vi "SUB_SFCS_SendResult.vi"(1 "ErrorCode":string, 2 "PASS_Fail (1/0)":i8) -> (0 "Sent OK ?":bool)   [LabVIEW 2011]
uses:
  Instance           4 27Saved   SUB_SFCS_SendResult .vi
  Instance           7 27Saved   SUB_SFCS_SendResult .vi
  Instance           8 27Saved   SUB_SFCS_SendResult .vi
  Instance          10 27Saved   SUB_SFCS_SendResult .vi
  Instance          11 27Saved   SUB_SFCS_SendResult .vi
  Instance          14 27Saved   SUB_SFCS_SendResult .vi
  Instance          15 27Saved   SUB_SFCS_SendResult .vi
  data/MCSDLL.dll
panel:
  out "output param":string
  out "SFCS System Enable":string
  out "OperatorID":string
  out "Line":string
  out "SN":string
  out "Station":string
  out "STAGE":string
  out "SFCS_IP":string
  in  "URL":string
  # "Send Result SFCS_Complete"
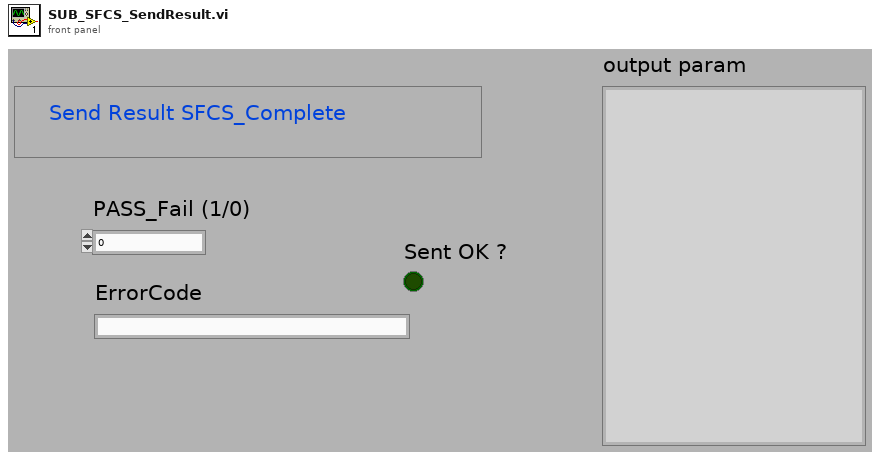
[diagram p1: front panel]
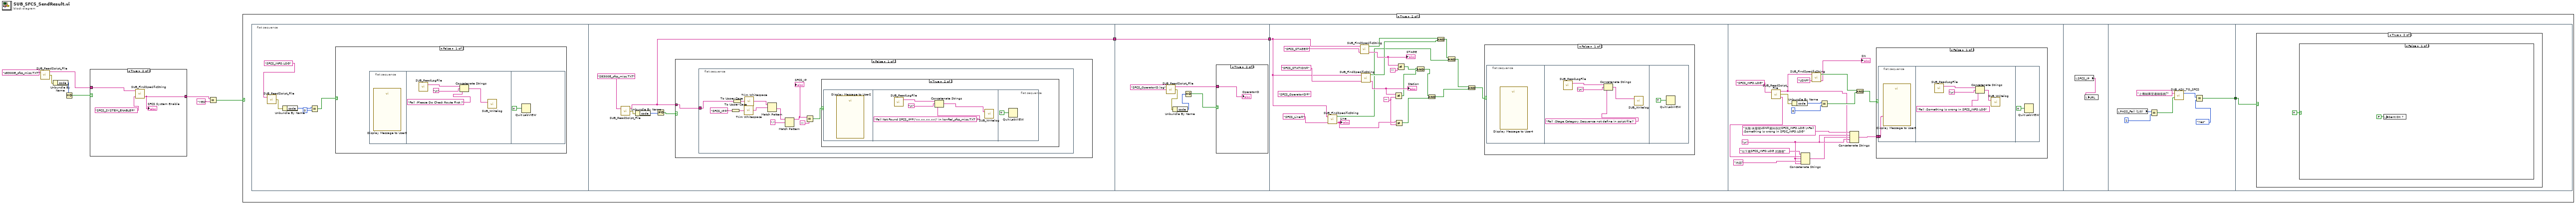
[diagram p0: block diagram]
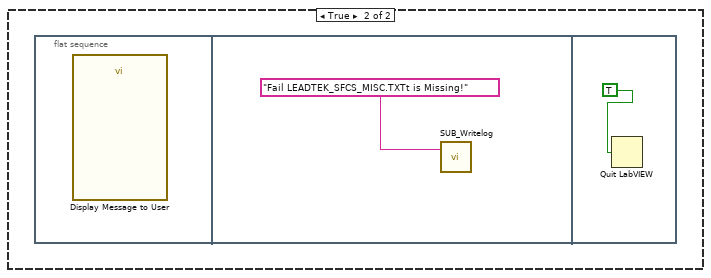
[diagram p5: hidden frame]
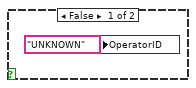
[diagram p6: hidden frame]
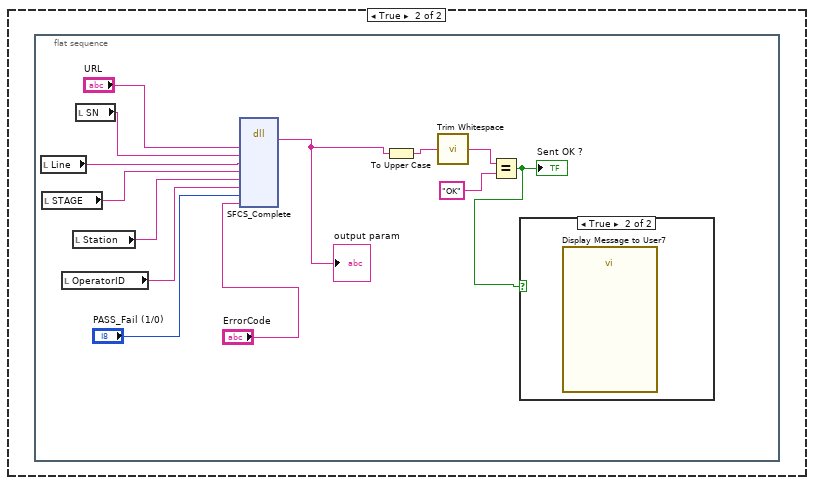
[diagram p10: hidden frame]
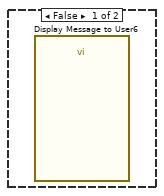
[diagram p11: hidden frame]
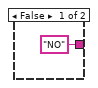
[diagram p12: hidden frame]
diagram:
  n1 = call "SUB_ReadScript_File.vi"("Script FileName"="s8300E_sfcs_misc.TXT") -> ("text"=w2:string, "error out"=w8:errorcluster)  [unwired: 1 in, 1 out]
  n2 = Unbundle By Name(w8) -> ("code"=w7:i32)
  n3 = Equal To 0?(x=w7) -> (x = 0?=w6:bool)
  n4 = case shown="True" w6 {
    tunnel: w2 -> [_ w12]
    tunnel: ["NO" ("before \"; \" string") w10] -> w4
    frame False {
    }
    frame True {
      n5 = call "SUB_FindSpecificString.vi"("Find this String"="SFCS_SYSTEM_ENABLE=", "String data"=w12) -> ("before \"; \" string"=w10:string)  [unwired: 2 in, 1 out]
      "SFCS System Enable" <- w10
    }
  }
  n6 = Equal?(x=w4, y="YES") -> (x = y?=w5:bool)
  n7 = case shown="True" w5 {
    frame False {
    }
    frame True {
      n8 = flat-sequence {
        tunnel: [w27] -> w14
        tunnel: w14 -> [w55]
        tunnel: [w55] -> w13
        tunnel: w13 -> [w73]
        tunnel: [w111] -> w15
        tunnel: w15 -> [w115]
        frame #0 {
          n9 = call "SUB_ReadScript_File.vi"("Script FileName"="SFCS_INFO.LOG" ("Search Filename in Folder")) -> ("error out"=w20:errorcluster)  [unwired: 1 in, 2 out]
          n10 = Unbundle By Name(w20) -> ("code"=w19:i32)
          n11 = Equal?(x=w19, y=0) -> (x = y?=w16:bool)
          n12 = case shown="False" w16 {
            frame False {
              n13 = flat-sequence {
                frame #0 {
                  n14 = call "Display Message to User3"() -> ()  [unwired: 10 in, 2 out]
                }
                frame #1 {
                  n15 = call "SUB_ReadLogFile.vi"() -> ("text"=w24:string)  [unwired: 2 in, 1 out]
                  n16 = Concatenate Strings(w24, "\n", "Fail :Please Do Check Route First !" ("Pass/Fail")) -> (w21:string)
                  n17 = call "SUB_Writelog.vi"("Pass/Fail"=w21) -> ()  [unwired: 2 in]
                }
                frame #2 {
                  n18 = Quit LabVIEW(quit? (T)=TRUE) -> ()
                }
              }
            }
            frame True {
            }
          }
        }
        frame #1 {
          n19 = call "SUB_ReadScript_File.vi"("Script FileName"="S8300E_sfcs_misc.TXT") -> ("text"=w27:string, "error out"=w30:errorcluster)  [unwired: 1 in, 1 out]
          n20 = Unbundle By Name(w30) -> ("code"=w29:i32)
          n21 = Not Equal To 0?(x=w29) -> (x != 0?=w28:bool)
          n22 = case shown="False" w28 {
            tunnel: w27 -> [w31 _]
            frame False {
              n23 = flat-sequence {
                tunnel: w31 -> [w37]
                frame #0 {
                  n24 = To Upper Case(1:"SFCS_IP=" ("string")) -> (0:w41:string)
                  n25 = To Upper Case(1:w37) -> (0:w42:string)
                  n26 = call <vilib>:"Trim Whitespace.vi"("string"=w41) -> ("trimmed string"=w39:string)  [unwired: 1 in]
                  n27 = call <vilib>:"Trim Whitespace.vi"("string"=w42) -> ("trimmed string"=w38:string)  [unwired: 1 in]
                  n28 = Match Pattern(string=w38, regular expression=w39) -> (after substring=w36:string)  [unwired: 1 in, 3 out]
                  n29 = Match Pattern(string=w36, regular expression=";") -> (before substring=w34:string)  [unwired: 1 in, 3 out]
                  "SFCS_IP" <- w34
                  n30 = Equal?(x=w34, y="") -> (x = y?=w32:bool)
                  n31 = case shown="True" w32 {
                    frame False {
                    }
                    frame True {
                      n32 = flat-sequence {
                        frame #0 {
                          n33 = call "Display Message to User2"() -> ()  [unwired: 10 in, 2 out]
                        }
                        frame #1 {
                          n34 = call "SUB_ReadLogFile.vi"() -> ("text"=w46:string)  [unwired: 2 in, 1 out]
                          n35 = Concatenate Strings(w46, "\n", "Fail Not Found SFCS_IP=\"xx.xx.xx.xx\" in konftel_sfcs_misc.TXT !" ("Pass/Fail")) -> (w43:string)
                          n36 = call "SUB_Writelog.vi"("Pass/Fail"=w43) -> ()  [unwired: 2 in]
                        }
                        frame #2 {
                          n37 = Quit LabVIEW(quit? (T)=TRUE) -> ()
                        }
                      }
                    }
                  }
                }
              }
            }
            frame True {
              n38 = flat-sequence {
                frame #0 {
                  n39 = call "Display Message to User"() -> ()  [unwired: 10 in, 2 out]
                }
                frame #1 {
                  n40 = call "SUB_Writelog.vi"("Pass/Fail"="Fail LEADTEK_SFCS_MISC.TXTt is Missing!") -> ()  [unwired: 2 in]
                }
                frame #2 {
                  n41 = Quit LabVIEW(quit? (T)=TRUE) -> ()
                }
              }
            }
          }
        }
        frame #2 {
          n42 = call "SUB_ReadScript_File.vi"("Script FileName"="SFCS_OperatorID.log" ("name or relative path")) -> ("text"=w50:string, "error out"=w53:errorcluster)  [unwired: 1 in, 1 out]
          n43 = Unbundle By Name(w53) -> ("code"=w52:i32)
          n44 = Equal To 0?(x=w52) -> (x = 0?=w51:bool)
          n45 = case shown="True" w51 {
            tunnel: w50 -> [_ w57]
            frame False {
              n46 = local write "OperatorID"("UNKNOWN" ("OperatorID")) -> ()
            }
            frame True {
              "OperatorID" <- w57
            }
          }
        }
        frame #3 {
          (unwired) "SFCS_OperatorID="
          w68 = ""
          n47 = call "SUB_FindSpecificString.vi"("Find this String"="SFCS_Line=", "String data"=w73) -> ("before \"; \" string"=w69:string, "Found"=w59:bool)  [unwired: 2 in]
          "Line" <- w69
          n48 = call "SUB_FindSpecificString.vi"("Find this String"="SFCS_STAGE=" ("string"), "String data"=w73) -> ("before \"; \" string"=w71:string, "Found"=w64:bool)  [unwired: 2 in]
          "STAGE" <- w71
          n49 = call "SUB_FindSpecificString.vi"("Find this String"="SFCS_STATION=" ("string"), "String data"=w73) -> ("before \"; \" string"=w70:string, "Found"=w63:bool)  [unwired: 2 in]
          "Station" <- w70
          n50 = Not Equal?(x=w70, y=w68) -> (x != y?=w66:bool)
          n51 = Not Equal?(x=w69, y=w68) -> (x != y?=w58:bool)
          n52 = Not Equal?(x=w71, y="") -> (x != y?=w67:bool)
          n53 = And(x=w67, y=w66) -> (x .and. y?=w65:bool)
          n54 = And(x=w65, y=w58) -> (x .and. y?=w60:bool)
          n55 = And(x=w64, y=w63) -> (x .and. y?=w62:bool)
          n56 = And(x=w62, y=w59) -> (x .and. y?=w61:bool)
          n57 = And(x=w61, y=w60) -> (x .and. y?=w76:bool)
          n58 = case shown="False" w76 {
            frame False {
              n59 = flat-sequence {
                frame #0 {
                  n60 = call "Display Message to User4"() -> ()  [unwired: 10 in, 2 out]
                }
                frame #1 {
                  n61 = call "SUB_ReadLogFile.vi"() -> ("text"=w81:string)  [unwired: 2 in, 1 out]
                  n62 = Concatenate Strings(w81, "\n", "Fail :Stage,Category,Sequence not define in script file!" ("Pass/Fail")) -> (w78:string)
                  n63 = call "SUB_Writelog.vi"("Pass/Fail"=w78) -> ()  [unwired: 2 in]
                }
                frame #2 {
                  n64 = Quit LabVIEW(quit? (T)=TRUE) -> ()
                }
              }
            }
            frame True {
            }
          }
        }
        frame #4 {
          w85 = "\n"
          n65 = call "SUB_ReadScript_File.vi"("Script FileName"="SFCS_INFO.LOG" ("name or relative path")) -> ("text"=w83:string, "error out"=w98:errorcluster, "path string"=w87:string)  [unwired: 1 in]
          n66 = Unbundle By Name(w98) -> ("code"=w96:i32)
          n67 = Concatenate Strings("以下是SFCS_INFO.LOG 於路徑", w87, w85, "內容", w85) -> (w84:string)
          n68 = call "SUB_FindSpecificString.vi"("Find this String"="USN=", "String data"=w83) -> ("before \"; \" string"=→"SN":string, "Found"=w92:bool)  [unwired: 2 in]
          n69 = Equal?(x=w96, y=0) -> (x = y?=w94:bool)
          n70 = Concatenate Strings("失敗:未發現USN=資料存於SFCS_INFO.LOG.\nFail :Something is wrong in SFSC_INFO.LOG", w85, w84, w85, w83) -> (w89:string)
          n71 = And(x=w92, y=w94) -> (x .and. y?=w93:bool)
          n72 = case shown="False" w93 {
            tunnel: w89 -> [w100 _]
            frame False {
              n73 = flat-sequence {
                tunnel: w100 -> [w101]
                frame #0 {
                  n74 = call "Display Message to User5"("Message"=w101) -> ()  [unwired: 9 in, 2 out]
                }
                frame #1 {
                  n75 = call "SUB_ReadLogFile.vi"() -> ("text"=w105:string)  [unwired: 2 in, 1 out]
                  n76 = Concatenate Strings(w105, "\n", "Fail :Something is wrong in SFCS_INFO.LOG" ("Pass/Fail")) -> (w102:string)
                  n77 = call "SUB_Writelog.vi"("Pass/Fail"=w102) -> ()  [unwired: 2 in]
                }
                frame #2 {
                  n78 = Quit LabVIEW(quit? (T)=TRUE) -> ()
                }
              }
            }
            frame True {
            }
          }
        }
        frame #5 {
          n79 = local read "SFCS_IP"() -> (w107:string)
          n80 = local write "URL"(w107) -> ()
        }
        frame #6 {
          n81 = local read "PASS_Fail (1/0)"() -> (w110:i8)
          n82 = Equal?(x=w110, y=i8 1) -> (x = y?=w108:bool)
          n83 = call "SUB_ASK_TO_SFCS.vi"("測試結果(報告)"=w108, "Question:"="上傳結果至遠端係統?") -> ("yes/no"=w113:enum32{"No Selection", "Yes", "No", "None"})  [unwired: 1 in]
          n84 = Equal?(x=w113, y=enum32{"No Selection", "Yes", "No", "None"}."Yes") -> (x = y?=w111:bool)
        }
        frame #7 {
          n85 = case shown="True" w115 {
            frame False {
            }
            frame True {
              n86 = case shown="False" TRUE {
                frame False {
                  n87 = local write "Sent OK ?"(FALSE ("Sent OK ?")) -> ()
                }
                frame True {
                  n88 = flat-sequence {
                    frame #0 {
                      n89 = local read "Line"() -> (w128:string)
                      n90 = local read "STAGE"() -> (w127:string)
                      n91 = local read "OperatorID"() -> (w125:string)
                      n92 = local read "Station"() -> (w126:string)
                      n93 = local read "SN"() -> (w129:string)
                      n94 = dll-call lib="D:/S8300E_Project/data/MCSDLL.dll" fn="SFCS_Complete"("URL"="URL", "SN"=w129, "Line"=w128, "Stage"=w127, "Station"=w126, "OperatorID"=w125, "PASS_Fail"="PASS_Fail (1/0)", "ErrorCode"="ErrorCode") -> (w122:string)  [unwired: 11 in, 2 out]
                      "output param" <- w122
                      n95 = To Upper Case(1:w122) -> (0:w123:string)
                      n96 = call <vilib>:"Trim Whitespace.vi"("string"=w123) -> ("trimmed string"=w121:string)  [unwired: 1 in]
                      n97 = Equal?(x=w121, y="OK") -> (x = y?=w119:bool)
                      "Sent OK ?" <- w119
                      n98 = case shown="True" w119 {
                        frame False {
                          n99 = call "Display Message to User6"() -> ()  [unwired: 10 in, 2 out]
                        }
                        frame True {
                          n100 = call "Display Message to User7"() -> ()  [unwired: 10 in, 2 out]
                        }
                      }
                    }
                  }
                }
              }
            }
          }
        }
      }
    }
  }
